vi "CE.vi"(7 "Number in":string, 8 "Error In":errorcluster, 9 "Unit scale In":string, 10 "Unit in":string, 11 "Decimal in":string) -> (0 "Error Out":errorcluster, 1 "Unit scale out":string, 2 "Unit out":string, 3 "Decimal out":string, 5 "Number out":string)   [LabVIEW 2021, in "Signal.lvlib"]
doc: "This subVI is used for deleting the keyboard string from right to left character by character."
uses:
  Signal.lvlib
panel:
  # "Input"
  # "Output"
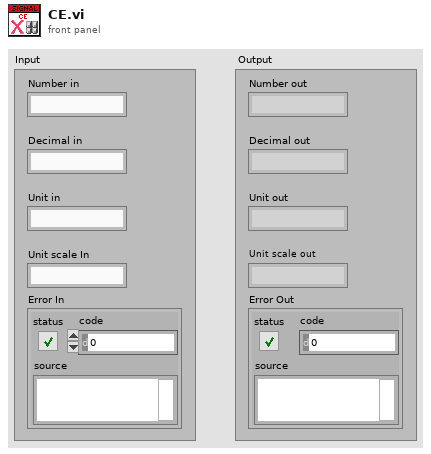
[diagram p1: front panel]
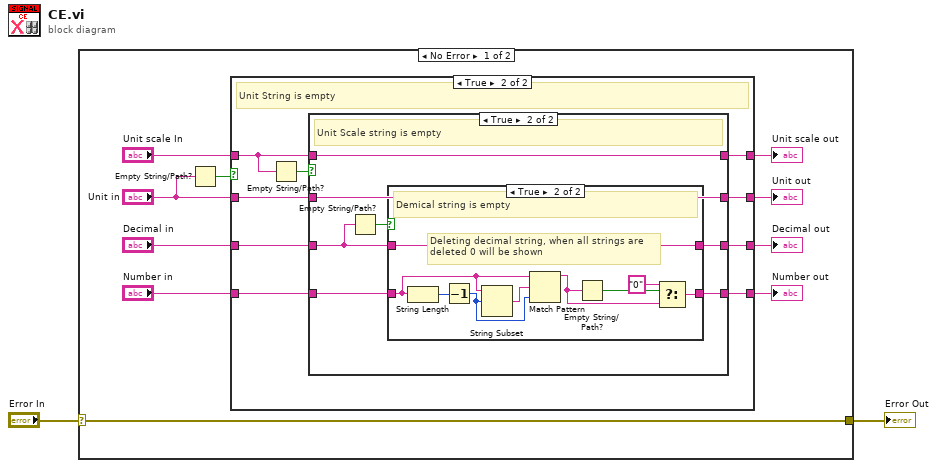
[diagram p0: block diagram]
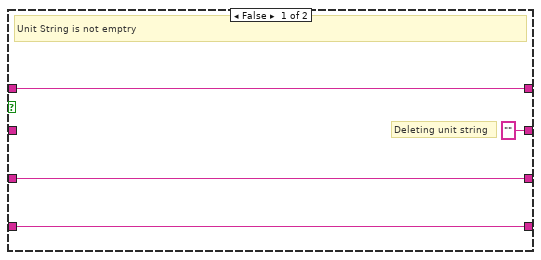
[diagram p2: hidden frame]
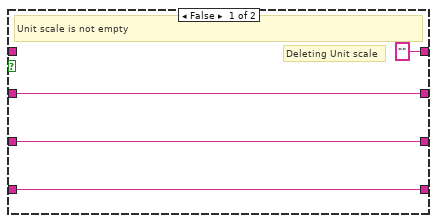
[diagram p3: hidden frame]
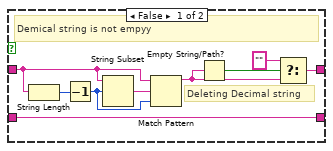
[diagram p4: hidden frame]
diagram:
  n1 = case shown="No Error" "Error In" {
    selector: "Error In" -> [w5 w55]
    tunnel: [w5 w55] -> w2
    frame No Error {
      n2 = Empty String/Path?(string/path="Unit in") -> (empty?=w4:bool)
      n3 = case shown="True" w4 {
        tunnel: "Decimal in" -> [w15 w25]
        tunnel: [w16 w24] -> w7
        tunnel: "Number in" -> [w16 w23]
        tunnel: [w15 w22] -> w9
        tunnel: ["" ("Unit in") w20] -> w10
        tunnel: [w14 w19] -> w12
        tunnel: "Unit scale In" -> [w14 w17]
        tunnel: "Unit in" -> [_ w21]
        frame False {
          # "Deleting unit string"
          # "Unit String is not emptry"
        }
        frame True {
          # "Unit String is empty"
          n4 = Empty String/Path?(string/path=w17) -> (empty?=w18:bool)
          n5 = case shown="True" w18 {
            tunnel: w25 -> [w28 w31]
            tunnel: [w29 w36] -> w24
            tunnel: w23 -> [w29 w35]
            tunnel: [w28 w34] -> w22
            tunnel: w21 -> [w27 w33]
            tunnel: [w27 w33] -> w20
            tunnel: w17 -> [_ w32]
            tunnel: ["" w32] -> w19
            frame False {
              # "Deleting Unit scale"
              # "Unit scale is not empty"
            }
            frame True {
              # "Unit Scale string is empty"
              n6 = Empty String/Path?(string/path=w31) -> (empty?=w30:bool)
              n7 = case shown="True" w30 {
                tunnel: w31 -> [w39 w54]
                tunnel: [w42 w49] -> w36
                tunnel: w35 -> [w42 w48]
                tunnel: [w40 w54] -> w34
                frame False {
                  # "Deleting Decimal string"
                  # "Demical string is not empyy"
                  n8 = String Length(string=w39) -> (length=w45:i32)
                  n9 = Decrement(x=w45) -> (x-1=w43:i32)
                  n10 = String Subset(string=w39, offset (0)=w43) -> (substring=w44:string)  [unwired: 1 in]
                  n11 = Match Pattern(string=w39, regular expression=w44, offset (0)=w43) -> (before substring=w38:string)  [unwired: 3 out]
                  n12 = Empty String/Path?(string/path=w38) -> (empty?=w37:bool)
                  n13 = Select(t="" ("y"), s=w37, f=w38) -> (s? t:f=w40:string)
                }
                frame True {
                  # "Deleting decimal string, when all strings are\ndeleted 0 will be shown"
                  # "Demical string is empty"
                  n14 = String Length(string=w48) -> (length=w53:i32)
                  n15 = Decrement(x=w53) -> (x-1=w51:i32)
                  n16 = String Subset(string=w48, offset (0)=w51) -> (substring=w52:string)  [unwired: 1 in]
                  n17 = Match Pattern(string=w48, regular expression=w52, offset (0)=w51) -> (before substring=w47:string)  [unwired: 3 out]
                  n18 = Empty String/Path?(string/path=w47) -> (empty?=w46:bool)
                  n19 = Select(t="0" ("y"), s=w46, f=w47) -> (s? t:f=w49:string)
                }
              }
            }
          }
        }
      }
      "Unit scale out" <- w12
      "Unit out" <- w10
      "Decimal out" <- w9
      "Number out" <- w7
    }
    frame Error {
    }
  }
  "Error Out" <- w2
